vi "NI PXI-4072 DMM RT Driver VI.vi"(6 "Device Clock":string, 9 "Device Inputs FIFO":refnum<k33>, 11 "Device Reference":T1 format="%.0x") -> ()   [LabVIEW 2010, in "NI PXI-4072 DMM Custom Device.lvlib"]
uses:
  NI PXI-4072 DMM Custom Device.lvlib
  <vilib>/NI VeriStand/Custom Device API/Custom Device Item Ref.ctl
  <vilib>/NI VeriStand/Custom Device API/Custom Device Channel Type.ctl
  <vilib>/Platform/TimedLoop/XDataNode/XDataNode.xnode
  <vilib>/Platform/TimedLoop/XDataNode/timing_clust.ctl
  <vilib>/Platform/TimedLoop/XDataNode/nitl_modes.ctl
  <vilib>/Platform/TimedLoop/XDataNode/wakeup.ctl
  <vilib>/NI VeriStand/Custom Device API/Get Item Property (I32).vi
  <vilib>/Platform/TimedLoop/XDataNode/XDNodeRunTimeDep.lvlib
  <vilib>/NI Veristand/Custom Device API/Custom Device API.lvlib
  <vilib>/NI Veristand/Custom Device Tools/Custom Device Utility Library/Custom Device Utility Library.lvlib
panel:
  in  "Device Outputs FIFO":refnum<k33>
  in  "Status Notifier":refnum<notifier>
  # "Custom Device Template\nv1.0"
  # "Use this template as a starting point for creating a custom device code module. The input controls shown here are specially named controls that the system will use to provide the device loop with data. The controls are not required for the device loop to run. For instance, if the device doesn't produce any output data, then you don't need the Device Outputs FIFO control. If you do use these controls, however, they need to have these exact names to be functional."
  # "The optional status notifier element is used to notify the RT engine of the last state of the custom device, and to indicate the device has completed execution. If this control is not used, a default No Error value is returned to the system when the device finishes execution.\n\nNote: This error state is not checked until the system shuts down. Use an output status channel to send more immediate status values to the system."
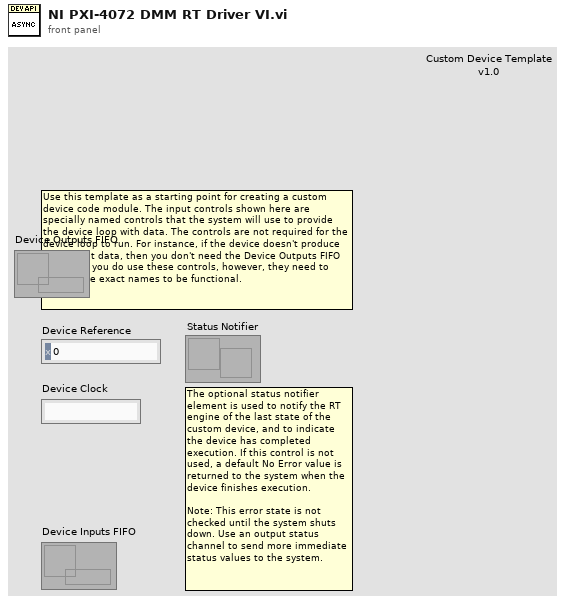
[diagram p1: front panel]
types:
  T1 = typedef "Custom Device API.lvlib/Custom Device Item Ref.ctl" = u64
  T2 = typedef "Custom Device API.lvlib/Custom Device Channel Type.ctl" = enum16{"Input", "Output"}
  T3 = typedef "Custom Device API.lvlib/Custom Device Timed Loop Priority.ctl" = enum32{"Low", "Medium", "High"}
  T4 = cluster{"instrument handle out":refnum<k15>, "Value":string, "Measurement Type":u16}
  T5 = typedef "XDNodeRunTimeDep.lvlib/timing_clust.ctl" = cluster{"Expected End [f-1]":u64, "Actual End [f-1]":u64, "Finished Late? [f-1]":bool, "Expected End [i-1]":u64, "Actual End [i-1]":u64, "Finished Late? [i-1]":bool, "Expected Start [i]":u64, "Actual Start [i]":u64, "Expected Start [f]":u64, "Actual Start [f]":u64, "Source Name":string, "Structure Name":string, "Period":i64, "Deadline":i64, "Offset":i64, "Start":i64, "Priority":i32, "Timeout":i32, "Mode":T6, "Wakeup Reason":T7, "Error":errorcluster, "Source Type":string, "Secondary Source Type":string, "Global End Time":u64, "Global Start Time":u64, "Frame Duration":u64, "Iteration Duration":u64, "Assigned CPU":i32, "I/O Scan Engine Mode":u32}
  T6 = typedef "XDNodeRunTimeDep.lvlib/nitl_modes.ctl" = enum32{"No Change", "Process missed periods, maintain original phase", "Discard missed periods, maintain original phase", "Process missed periods, ignore original phase", "Discard missed periods, ignore original phase"}
  T7 = typedef "XDNodeRunTimeDep.lvlib/wakeup.ctl" = enum32{"Normal", "Aborted", "Asynchronous wakeup", "Timing source error", "Timed loop error", "Timeout"}
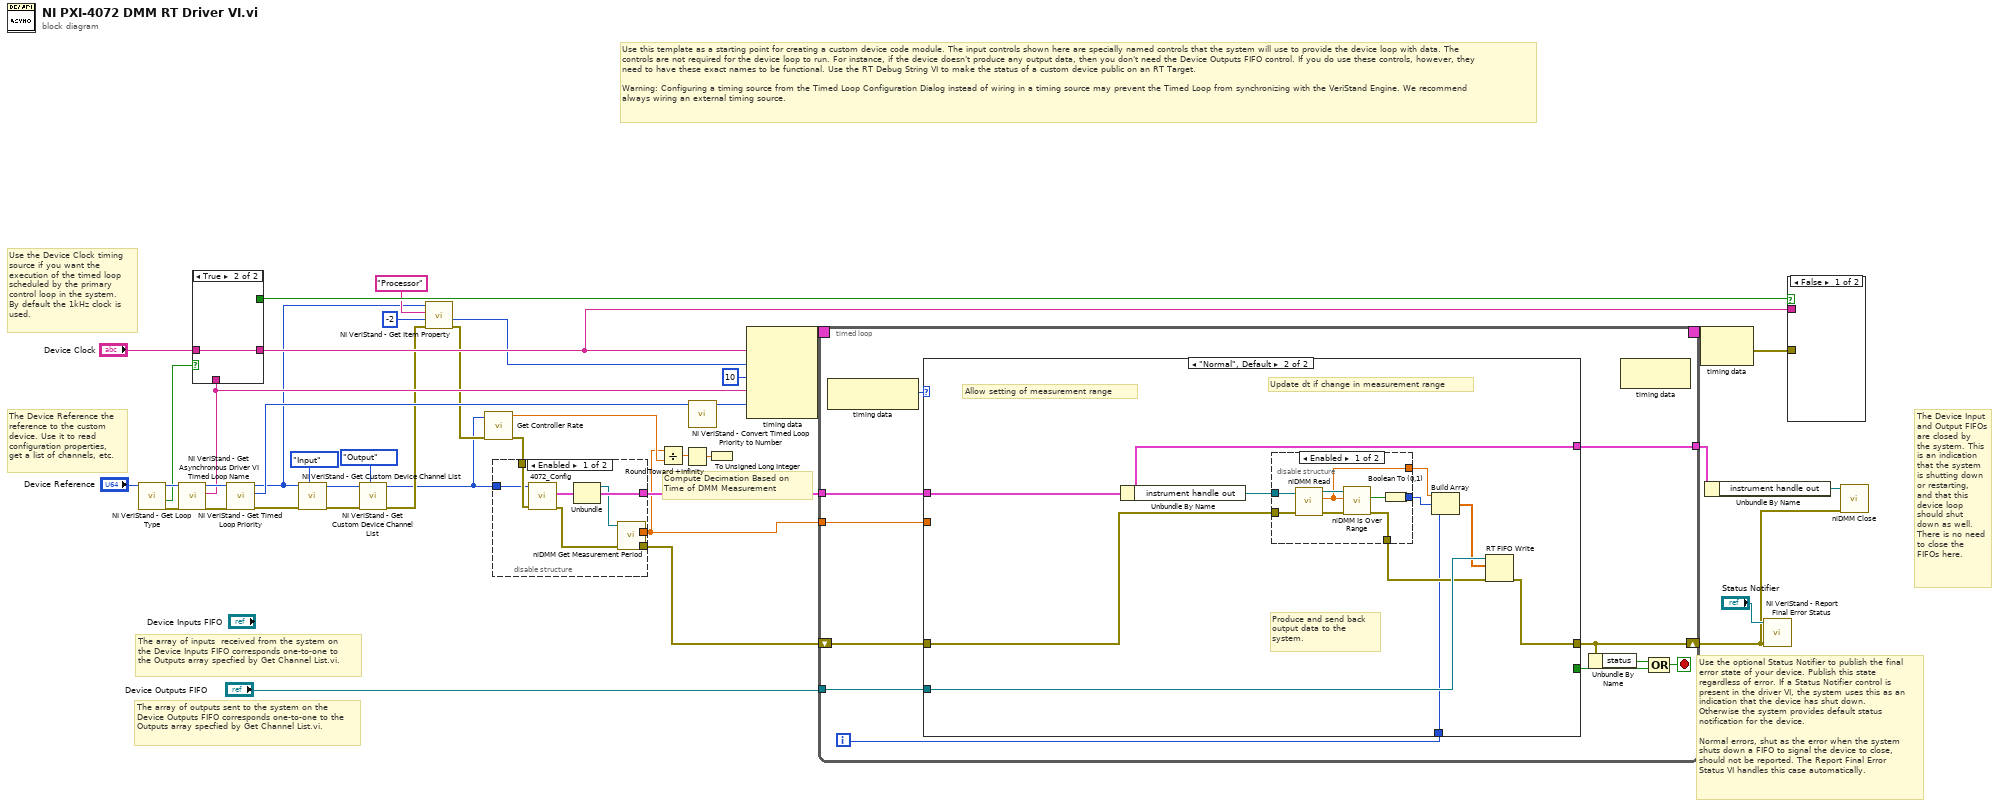
[diagram p0: block diagram]
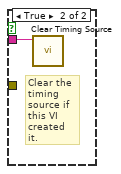
[diagram p3: hidden frame]
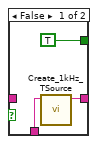
[diagram p4: hidden frame]
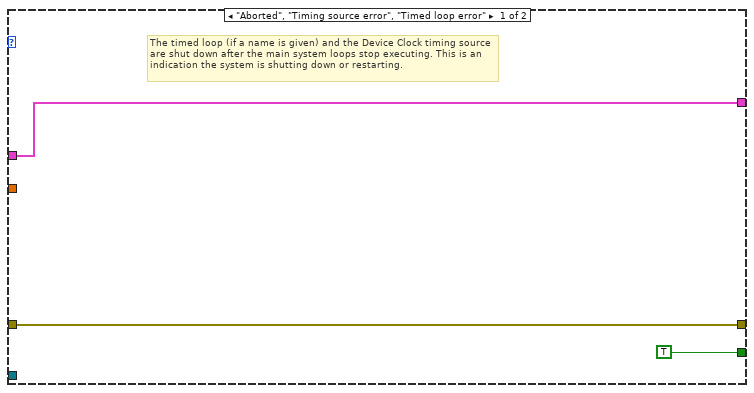
[diagram p5: hidden frame]
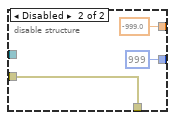
[diagram p6: hidden frame]
diagram:
  # "Compute Decimation Based on\nTime of DMM Measurement"
  # "The array of inputs  received from the system on the Device Inputs FIFO corresponds one-to-one to the Outputs array specfied by Get Channel List.vi."
  # "Use the optional Status Notifier to publish the final error state of your device. Publish this state regardless of error. If a Status Notifier control is present in the driver VI, the system uses this as an indication that the device has shut down. Otherwise the system provides default status notification for the device.\n\nNormal errors, shut as the error when the system shuts down a FIFO to signal the device to close, should not be reported. The Report Final Error Status VI handles this case automatically."
  # "The Device Input and Output FIFOs are closed by the system. This is an indication that the system is shutting down or restarting, and that this device loop should shut down as well. There is no need to close the FIFOs here."
  # "The array of outputs sent to the system on the Device Outputs FIFO corresponds one-to-one to the Outputs array specfied by Get Channel List.vi."
  # "The Device Reference the reference to the custom device. Use it to read configuration properties, get a list of channels, etc."
  # "Use the Device Clock timing source if you want the execution of the timed loop scheduled by the primary control loop in the system. \nBy default the 1kHz clock is used."
  # "Use this template as a starting point for creating a custom device code module. The input controls shown here are specially named controls that the system will use to provide the device loop with data. The controls are not required for the device loop to run. For instance, if the device doesn't produce any output data, then you don't need the Device Outputs FIFO control. If you do use these controls, however, they need to have these exact names to be functional. Use the RT Debug String VI to make the status of a custom device public on an RT Target.\n\nWarning: Configuring a timing source from the Timed Loop Configuration Dialog instead of wiring in a timing source may prevent the Timed Loop from synchronizing with the VeriStand Engine. We recommend always wiring an external timing source."
  n1 = call <vilib>:"NI VeriStand - Get Loop Type.vi"("Device Ref in"="Device Reference") -> ("error out"=w34:errorcluster, "Use Device Clock"=w32:bool, "Device Ref out"=w33:T1)  [unwired: 1 in, 7 out]
  n2 = call <vilib>:"NI VeriStand - Get Asynchronous Driver VI Timed Loop Name.vi"("error in (no error)"=w34, "Device Ref in"=w33) -> ("error out"=w37:errorcluster, "Device Timed Loop Name"=w26:string, "Device Ref out"=w40:T1)  [unwired: 7 out]
  n3 = case shown="True" w32 {
    tunnel: "Device Clock" -> [_ w44]
    tunnel: [w43 w44] -> w27
    tunnel: [TRUE _] -> w28
    tunnel: w26 -> [w41 _]
    frame False {
      n4 = call <vilib>:"Create_1kHz_TSource.vi"("name (in)"=w41) -> ("name (out)"=w43:string)  [unwired: 1 in, 9 out]
    }
    frame True {
    }
  }
  n5 = call <vilib>:"NI VeriStand - Get Timed Loop Priority.vi"("error in (no error)"=w37, "Device Ref in"=w40) -> ("error out"=w24:errorcluster, "Priority"=w36:T3, "Device Ref out"=w12:T1)  [unwired: 7 out]
  n6 = call <vilib>:"NI VeriStand - Get Custom Device Channel List.vi"("Channel Type"=Custom_Device_Channel_Type."Input", "error in (no error)"=w24, "Device Ref in"=w12) -> ("error out"=w18:errorcluster, "Device Ref out"=w19:T1)  [unwired: 7 out]
  n7 = call <vilib>:"NI VeriStand - Get Custom Device Channel List.vi"("Channel Type"=Custom_Device_Channel_Type."Output", "error in (no error)"=w18, "Device Ref in"=w19) -> ("error out"=w11:errorcluster, "Device Ref out"=w6:T1)  [unwired: 7 out]
  n8 = call-poly <vilib>:"NI VeriStand - Get Item Property.vi"("error in (no error)"=w11, "Default Value"=-2, "Property Name"="Processor", "Item Ref in"=w12) -> ("error out"=w7:errorcluster, "Value"=w16:i32)  [unwired: 4 in, 2 out]
  n9 = call "Get Controller Rate.vi"("error in (no error)"=w7, "Device Reference In"=w6) -> ("error out"=w8:errorcluster, "System dt in Secs"=w4:dbl)  [unwired: 7 in, 1 out]
  n10 = disable-structure shown="Enabled" {
    disable-tunnel: [w51 _] -> w10
    disable-tunnel: [w48 w52] -> w9
    disable-tunnel: w8 -> [w47 w52]
    disable-tunnel: w6 -> [w46 _]
    disable-tunnel: [w45 _] -> w2
    frame Enabled {
      n11 = call "4072_Config.vi"("error in (no error)"=w47, "Device Ref out"=w46) -> ("error out"=w49:errorcluster, "Instrument Handle Out"=w51:T4)  [unwired: 8 in]
      n12 = Unbundle(w51) -> ("instrument handle out"=w50:refnum<k15>)  [unwired: 2 out]
      n13 = call <instrlib>:"niDMM Get Measurement Period.vi"("error in (no error)"=w49, "instrument handle"=w50) -> ("error out"=w48:errorcluster, "Measurement Period (seconds)"=w45:dbl)  [unwired: 7 in, 1 out]
    }
    frame Disabled {
    }
  }
  n14 = Divide(x=w2, y=w4) -> (x/y=w5:dbl)
  n15 = Round Toward +Infinity(x=w5) -> (ceil(x): smallest int >= x=w3:dbl)
  n16 = call <vilib>:"NI VeriStand - Convert Timed Loop Priority to Number.vi"("Priority"=w36) -> ("Numeric Priority"=w35:i32)  [unwired: 10 out]
  n17 = To Unsigned Long Integer(number=w3) -> ()  [unwired: 1 out]
  n18 = node-c288(w27, w16, i64 10 ("Period"), w26, w35) -> (w39:T5)
  n19 = timed-loop {
    timing: w39 -> [_]
    timing-out: [_] -> w38
    shift-right: [w56] -> w23
    shift-left: w9 -> [w63]
    tunnel: w10 -> [w58]
    tunnel: [w57] -> w22
    tunnel: "Device Outputs FIFO" -> [w55]
    tunnel: w2 -> [w54]
    i -> [w53]
    stop <- w59 stop-if-true
    n20 = node-c288() -> (w62:T7)  [unwired: 1 out]
    n21 = case shown="\"Normal\", Default" w62 {
      tunnel: w63 -> [w67 w69]
      tunnel: [w67 w72] -> w56
      tunnel: [TRUE _] -> w60
      tunnel: w58 -> [w65 w77]
      tunnel: [w65 w77] -> w57
      tunnel: w55 -> [_ w74]
      tunnel: w54 -> [_ _]
      tunnel: w53 -> [_ w68]
      frame "Aborted", "Timing source error", "Timed loop error" {
        # "The timed loop (if a name is given) and the Device Clock timing source are shut down after the main system loops stop executing. This is an indication the system is shutting down or restarting."
      }
      frame "Normal", Default {
        # "Allow setting of measurement range"
        # "Update dt if change in measurement range"
        # "Produce and send back output data to the system."
        n22 = Unbundle By Name(w77) -> ("instrument handle out"=w70:refnum<k15>)
        n23 = disable-structure shown="Enabled" {
          disable-tunnel: [w82 -999.0 ("Measurement")] -> w76
          disable-tunnel: [w81 i16 999] -> w75
          disable-tunnel: [w80 w88] -> w73
          disable-tunnel: w70 -> [w79 _]
          disable-tunnel: w69 -> [w78 w88]
          frame Enabled {
            n24 = call <instrlib>:"niDMM Read.vi"("error in (no error)"=w78, "instrument handle"=w79) -> ("error out"=w84:errorcluster, "Measurement"=w82:dbl, "instrument handle out"=w85:refnum<k15>)  [unwired: 7 in]
            n25 = call <instrlib>:"niDMM Is Over Range.vi"("error in (no error)"=w84, "Measurement"=w82, "instrument handle"=w85) -> ("error out"=w80:errorcluster, "Over Range?"=w83:bool)  [unwired: 6 in, 1 out]
            n26 = Boolean To (0,1)(Boolean=w83) -> (0, 1=w81:i16)
          }
          frame Disabled {
          }
        }
        n27 = Build Array(w76, w75, w68) -> (w71:dbl[])
        n28 = RT FIFO Write(0:w74, 1:w71, 3:w73) -> (11:w72:errorcluster)  [unwired: 2 in, 3 out]
      }
    }
    n29 = Unbundle By Name(w56) -> ("status"=w61:bool)
    n30 = node-c288() -> ()  [unwired: 2 out]
    n31 = Compound Arithmetic op=OR(w61, w60) -> (w59:bool)
  }
  n32 = node-c288(w38) -> (w29:errorcluster)
  n33 = Unbundle By Name(w22) -> ("instrument handle out"=w21:refnum<k15>)
  n34 = call <vilib>:"NI VeriStand - Report Final Error Status.vi"("error in (no error)"=w23, "Status Notifier"="Status Notifier") -> ()  [unwired: 1 in, 9 out]
  n35 = case shown="False" w28 {
    tunnel: w29 -> [_ _]
    tunnel: w27 -> [_ w91]
    frame False {
    }
    frame True {
      # "Clear the timing source if this VI created it."
      n36 = call <vilib>:"Clear Timing Source.vi"("name"=w91) -> ()  [unwired: 1 in, 10 out]
    }
  }
  n37 = call <instrlib>:"niDMM Close.vi"("error in (no error)"=w23, "instrument handle"=w21) -> ()  [unwired: 9 in, 1 out]
